vi "tm_setinputtrigger_41.vi"(8 "error in (no error)":errorcluster, 9 "Options":T1={"Polarity"=1, "Times"=1, "Delay"=0.0} {"Polarity" items=["Negative"=1, "Positive"=2]}, 10 "Parameters":cluster{"Source":i32, "Active":i32, "Mode":i32}={"Source"=1, "Active"=1, "Mode"=1} {"Mode" items=["Normal"=1, "PIV"=3, "Start Trigger"=6, "Multigate"=7, "Multiframe"=8]; "Active" items=["Edge"=1, "Level"=2, "Sync Readout"=3, "Point"=4]; "Source" items=["Internal"=1, "External"=2, "Software"=3, "Master Pulse"=4]}, 11 "Handle in":u32) -> (0 "error out":errorcluster, 3 "Handle out":u32)   [LabVIEW 2023]
uses:
  tmcamcon.dll
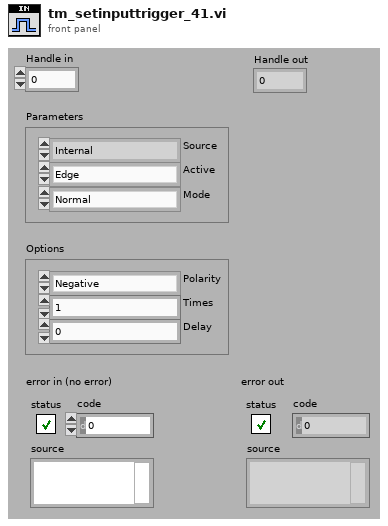
[diagram p1: front panel]
types:
  T1 = cluster{"Polarity":i32, "Times":i32, "Delay":dbl}
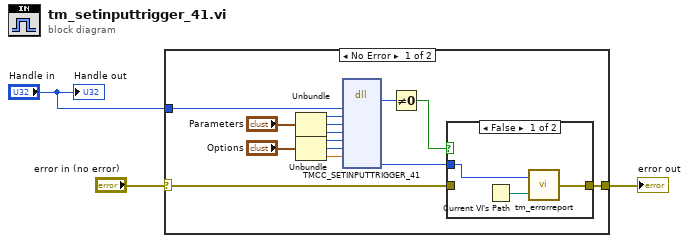
[diagram p0: block diagram]
diagram:
  n1 = case shown="No Error" "error in (no error)" {
    selector: "error in (no error)" -> [w15 w22]
    tunnel: [w12 w22] -> w2
    tunnel: "Handle in" -> [w16 _]
    frame No Error {
      n2 = Unbundle("Parameters") -> ("Source"=w9:i32, "Active"=w8:i32, "Mode"=w7:i32)
      n3 = Unbundle("Options") -> ("Polarity"=w6:i32, "Times"=w5:i32, "Delay"=w4:dbl)
      n4 = dll-call lib="tmcamcon.dll" fn="TMCC_SETINPUTTRIGGER_41"("HDCAM"=w16, "source"=w9, "active"=w8, "mode"=w7, "polarity"=w6, "times"=w5, "delay"=w4) -> ("return type"=w17:u32, "Erval"=w14:i32)  [unwired: 11 in, 2 out]
      n5 = Not Equal To 0?(x=w17) -> (x != 0?=w13:bool)
      n6 = case shown="False" w13 {
        tunnel: w15 -> [_ w21]
        tunnel: [w19 w21] -> w12
        tunnel: w14 -> [w18 _]
        frame False {
          n7 = Current VI's Path() -> (path=w20:path)
          n8 = call "tm_errorreport.vi"("Source"=w20, "Error"=w18) -> ("error out"=w19:errorcluster)
        }
        frame True {
        }
      }
    }
    frame Error {
    }
  }
  "error out" <- w2
  "Handle out" <- "Handle in"
